vi "SaveAndDisplayRsh.vi"(9 "Array":dbl[](array[numeric]), 10 "array":dbl[][](array[numeric]), 11 "file path (csv write)":path) -> (2 "output array":dbl[][](array[numeric]), 3 "XY Graph 4":cluster{"array":dbl[], "array":dbl[]}(graph))   [LabVIEW 2017]
uses:
  <vilib>/Utility/file.llb/Write Delimited Spreadsheet (DBL).vi
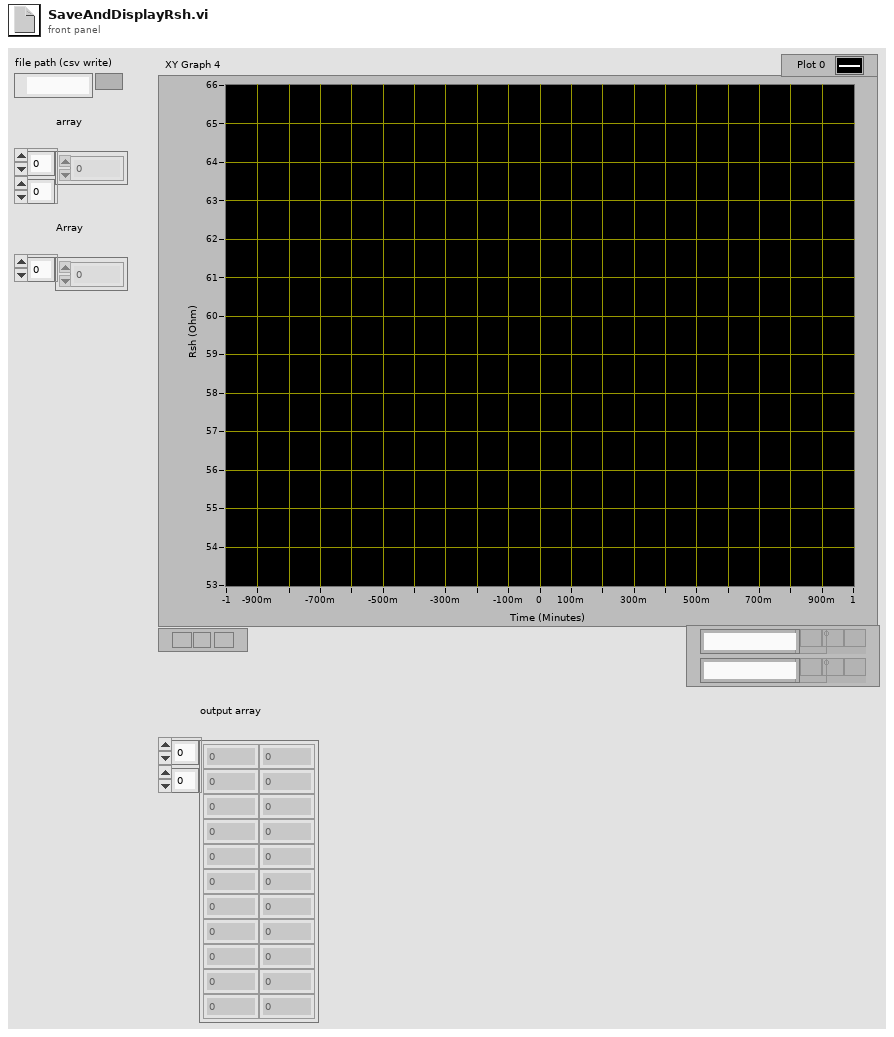
[diagram p1: front panel]
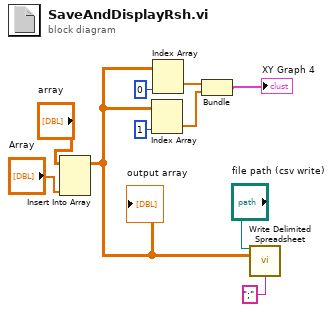
[diagram p0: block diagram]
diagram:
  n1 = Insert Into Array(array="array", new element="Array") -> (w10:dbl[][])  [unwired: 2 in]
  "output array" <- w10
  n2 = Index Array(array=w10, index (col)=1 ("disabled index (col)")) -> (element=w7:dbl[])  [unwired: 1 in]
  n3 = Index Array(array=w10, index (col)=0 ("disabled index (col)")) -> (element=w6:dbl[])  [unwired: 1 in]
  n4 = Bundle("array"=w6, "array"=w7) -> (→"XY Graph 4":cluster{"array":dbl[], "array":dbl[]})  [unwired: 1 in]
  n5 = call-poly <vilib>:"Write Delimited Spreadsheet.vi"("file path (dialog if empty)"="file path (csv write)", "2D data"=w10, "delimiter (\\t)"=";" ("delimiter (\\t)")) -> ()  [unwired: 11 in, 2 out]
